vi "week6_while_loops_LV17.vi"() -> ()   [LabVIEW 2017]
panel:
  out "Iteration 5":dbl
  out "Iteration 4":dbl
  out "Iteration 3 local variable":dbl
  out "Iteration 3 notification":dbl
  in  "SEND":bool
  out "XY Graph":cluster{"Y":dbl[], "Y":dbl[]}[](graph)
  out "Iteration 3":dbl
  out "Iteration 2":dbl
  out "Iteration 1":dbl
  in  "Rate 3 (sec)":dbl=3.0
  in  "Rate 2 (sec)":dbl=1.0
  in  "Rate 1 (sec)":dbl=2.0
  in  "Stop 3":bool
  in  "Stop 2":bool
  in  "Stop 1":bool
  in  "STOP ALL":bool
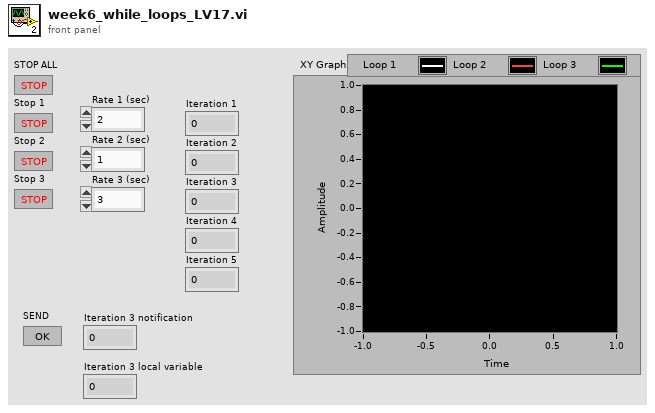
[diagram p1: front panel]
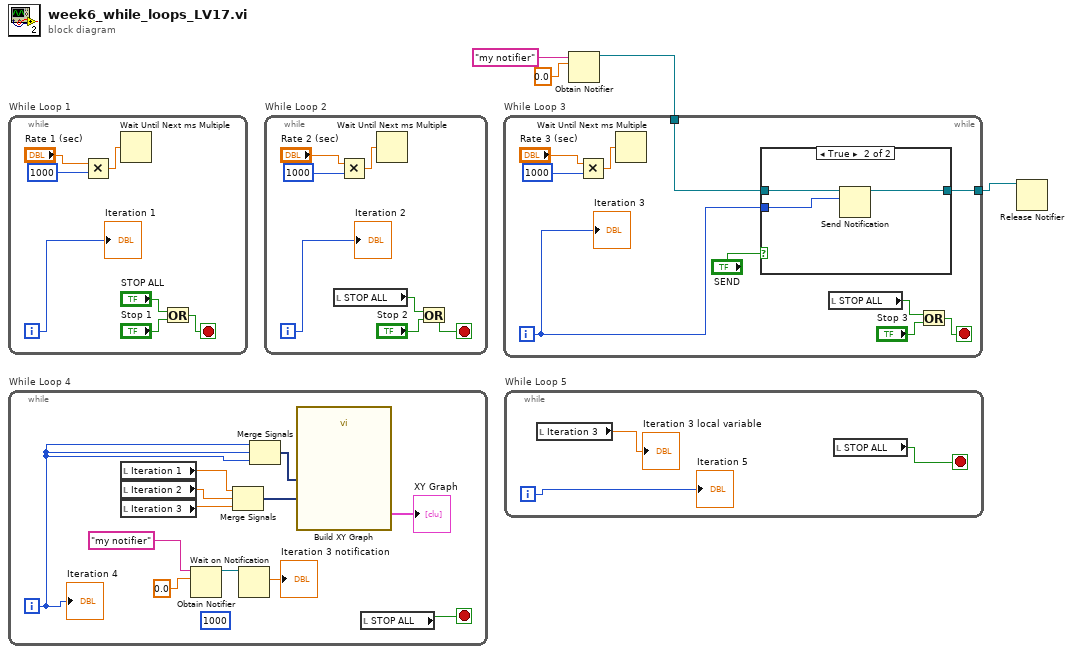
[diagram p0: block diagram]
diagram:
  n1 = while "While Loop 1" {
    i -> [w5]
    stop <- w9 stop-if-true
    n2 = Multiply(x="Rate 1 (sec)", y=1000) -> (x*y=w8:dbl)
    n3 = Wait Until Next ms Multiple(millisecond multiple=w8) -> ()  [unwired: 1 out]
    n4 = Or(x="STOP ALL", y="Stop 1") -> (x .or. y?=w9:bool)
    "Iteration 1" <- w5
  }
  n5 = while "While Loop 4" {
    i -> [w12]
    stop <- w23 stop-if-true
    (unwired) 1000
    n6 = local read "Iteration 1"() -> (w18:dbl)
    n7 = local read "Iteration 2"() -> (w19:dbl)
    n8 = local read "Iteration 3"() -> (w20:dbl)
    n9 = Obtain Notifier(name (unnamed)="my notifier", notification data type=0.0) -> (notifier out=w15:refnum<notifier>)  [unwired: 2 in, 2 out]
    n10 = Merge Signals(w18, w19, w20) -> (w21:dynamicdata)
    n11 = Wait on Notification(notifier=w15) -> (notification=→"Iteration 3 notification":dbl)  [unwired: 3 in, 3 out]
    n12 = Merge Signals(w12, w12, w12) -> (w17:dynamicdata)
    n13 = call "Build XY Graph"("Y Input"=w21, "X Input"=w17) -> ("XY Graph"=→"XY Graph":cluster{"X":dbl[], "Y":dbl[]}[])  [unwired: 8 in, 1 out]
    n14 = local read "STOP ALL"() -> (w23:bool)
    "Iteration 4" <- w12
  }
  n15 = while "While Loop 2" {
    i -> [w24]
    stop <- w30 stop-if-true
    n16 = local read "STOP ALL"() -> (w28:bool)
    n17 = Multiply(x="Rate 2 (sec)", y=1000) -> (x*y=w27:dbl)
    n18 = Wait Until Next ms Multiple(millisecond multiple=w27) -> ()  [unwired: 1 out]
    n19 = Or(x=w28, y="Stop 2") -> (x .or. y?=w30:bool)
    "Iteration 2" <- w24
  }
  n20 = while "While Loop 5" {
    i -> [w31]
    stop <- w33 stop-if-true
    n21 = local read "Iteration 3"() -> (→"Iteration 3 local variable":dbl)
    n22 = local read "STOP ALL"() -> (w33:bool)
    "Iteration 5" <- w31
  }
  n23 = Obtain Notifier(name (unnamed)="my notifier", notification data type=0.0) -> (notifier out=w3:refnum<notifier>)  [unwired: 2 in, 2 out]
  n24 = while "While Loop 3" {
    tunnel: w3 -> [w35]
    tunnel: [w36] -> w2
    i -> [w37]
    stop <- w43 stop-if-true
    n25 = Multiply(x="Rate 3 (sec)", y=1000) -> (x*y=w40:dbl)
    n26 = Wait Until Next ms Multiple(millisecond multiple=w40) -> ()  [unwired: 1 out]
    n27 = case shown="True" "SEND" {
      tunnel: w37 -> [_ w47]
      tunnel: [w44 w46] -> w36
      tunnel: w35 -> [w44 w45]
      frame False {
      }
      frame True {
        n28 = Send Notification(notification=w47, notifier=w45) -> (notifier out=w46:refnum<notifier>)  [unwired: 1 in, 1 out]
      }
    }
    n29 = local read "STOP ALL"() -> (w41:bool)
    n30 = Or(x=w41, y="Stop 3") -> (x .or. y?=w43:bool)
    "Iteration 3" <- w37
  }
  n31 = Release Notifier(notifier=w2) -> ()  [unwired: 2 in, 3 out]
